vi "3D_Stem_Plot_Merge_VI.vi"() -> ()   [LabVIEW 2017]
uses:
  <vilib>/Math Plots/3D Math Plots/3D Stem/3D Stem XCtrl/3D Stem.xctl
  <vilib>/Math Plots/3D Math Plots/3D Stem/3D Stem Datatype/Public/Plot Helper (Vector).vi
  <vilib>/Math Plots/3D Math Plots/3D Stem/3D Stem Datatype/3D Stem Datatype.lvclass
panel:
  out "3D Stem":refnum<class "3D Plot Datatype.lvclass">[](xcontrol)
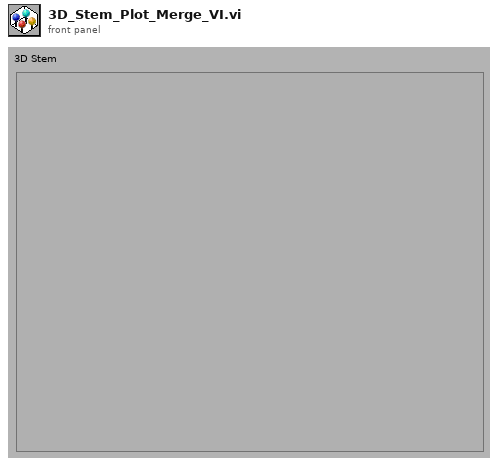
[diagram p1: front panel]
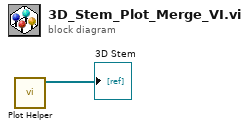
[diagram p0: block diagram]
diagram:
  n1 = call-poly <vilib>:"Plot Helper.vi"() -> ("3D Plot lvclass Array out"=→"3D Stem":refnum<class "3D Plot Datatype.lvclass">[])  [unwired: 6 in, 5 out]
